vi "Parse Error Response.vi"(5 "Error String":string) -> (6 "error code":i32, 8 "error message":string)   [LabVIEW 2013]
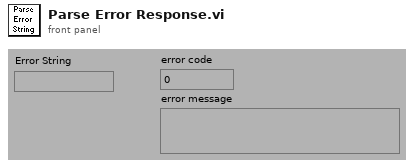
[diagram p1: front panel]
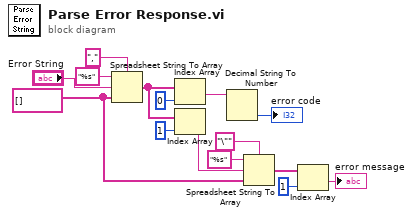
[diagram p0: block diagram]
diagram:
  w5 = string[] []
  n1 = Spreadsheet String To Array(delimiter (Tab)=",", format string="%s", spreadsheet string="Error String", array type (2D Dbl)=w5) -> (array=w9:string[])
  n2 = Index Array(array=w9, index=0) -> (element=w11:string)
  n3 = Index Array(array=w9, index=1) -> (element=w4:string)
  n4 = Decimal String To Number(string=w11) -> (number=→"error code":i32)  [unwired: 3 out]
  n5 = Spreadsheet String To Array(delimiter (Tab)="\"", format string="%s", spreadsheet string=w4, array type (2D Dbl)=w5) -> (array=w3:string[])
  n6 = Index Array(array=w3, index=1) -> (element=→"error message":string)
